vi "Load Module.vi"(8 "error in":errorcluster, 11 "Config Section":string) -> (0 "error out":errorcluster, 3 "Module ID (dup)":i32)   [LabVIEW 2014, in "DB_CONNECTOR.lvlib"]
uses:
  DB_CONNECTOR.lvlib
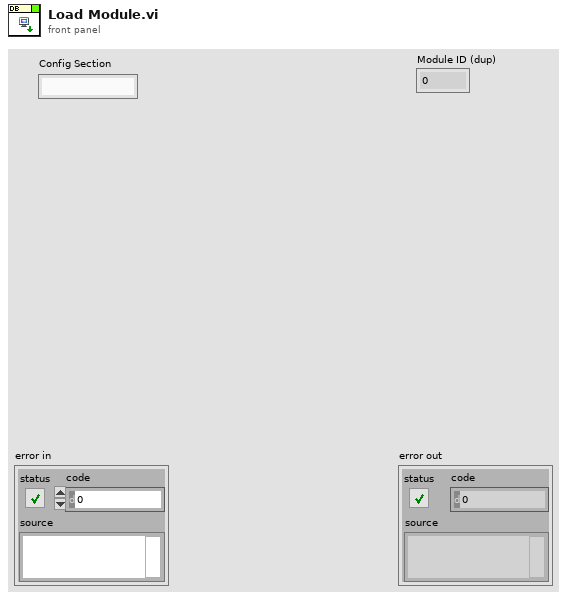
[diagram p1: front panel]
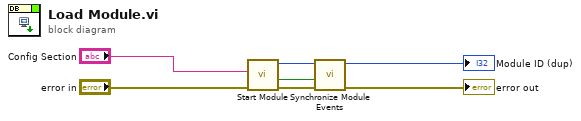
[diagram p0: block diagram]
diagram:
  n1 = call "Start Module.vi"("error in (no error)"="error in", "Config Section"="Config Section") -> ("error out"=w6:errorcluster, "Wait for Event Sync?"=w7:bool, "Module ID"=w5:i32)  [unwired: 6 in, 1 out]
  n2 = call "Synchronize Module Events.vi"("error in (no error)"=w6, "Wait for Event Sync?"=w7, "Module ID"=w5) -> ("error out"=→"error out":errorcluster, "Module ID (dup)"=→"Module ID (dup)":i32)  [unwired: 7 in]
